vi "Thar.vi"() -> ()   [LabVIEW 2016]
panel:
  in  "configuration file path":path
  out "error out":errorcluster
  in  "error in (no error)":errorcluster
  in  "stop":bool
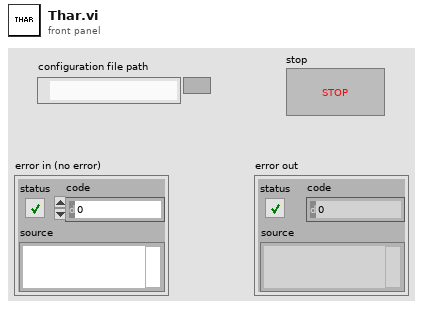
[diagram p1: front panel]
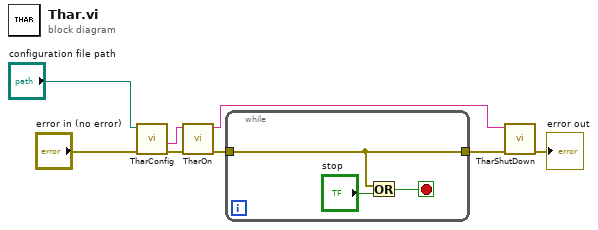
[diagram p0: block diagram]
diagram:
  n1 = call "TharConfig.vi"("Error In"="error in (no error)", "configuration file path"="configuration file path") -> ("Error Out"=w3:errorcluster, "serial"=w4:string)  [unwired: 6 in, 2 out]
  n2 = call "TharOn.vi"("Error In"=w3, "Device Serial Number"=w4) -> ("Error Out"=w7:errorcluster, "Device Serial Number Out"=w5:string)  [unwired: 8 in]
  n3 = while {
    tunnel: w7 -> [w9]
    tunnel: [w9] -> w6
    stop <- w10 stop-if-true
    n4 = Or(x=w9, y="stop") -> (x .or. y?=w10:bool)
  }
  n5 = call "TharShutDown.vi"("error in (no error)"=w6, "Device Serial Number"=w5) -> ("Error Out"=→"error out":errorcluster)  [unwired: 8 in, 1 out]
